vi "VFDRxClearLoop.vi"   [LabVIEW 2018]
uses:
  <vilib>/rvi/DataTransferAndStorage/Container/XNode/niFpgaContainer.xnode
  <vilib>/eio/EIOMethodNode/EIOMethodNode.xnode
  <vilib>/rvi/eio/common/nirviEmuTemplateMethod_errors.vi
  <vilib>/rvi/FIFO/Fifo_Resource/nirvififoEmulationClear.vi
  <vilib>/rvi/FIFO/Fifo_Resource/nirvififoEmulationRead.vi
  <vilib>/rvi/FIFO/Fifo_Resource/nirvififoEmulationWrite.vi
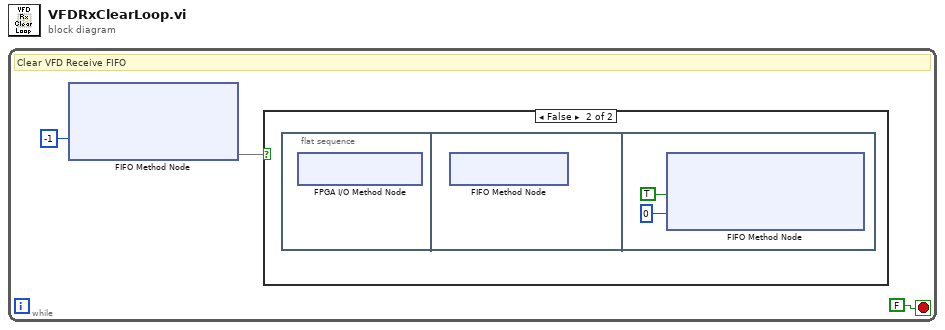
[diagram p0: block diagram]
diagram:
  n1 = while {
    stop <- FALSE stop-if-true
    # "Clear VFD Receive FIFO"
    n2 = xnode ("FIFO Method Node")("Timeout"=-1) -> ("Timed Out?"=w1)  [unwired: 1 in, 2 out]
    n3 = case shown="False" w1 {
      frame True {
      }
      frame False {
        n4 = flat-sequence {
          frame #0 {
            n5 = xnode "FPGA I/O Method Node"() -> ()  [unwired: 1 in, 1 out]
          }
          frame #1 {
            n6 = xnode ("FIFO Method Node")() -> ()  [unwired: 1 in, 1 out]
          }
          frame #2 {
            n7 = xnode ("FIFO Method Node")("Element"=TRUE, "Timeout"=0) -> ()  [unwired: 1 in, 2 out]
          }
        }
      }
    }
  }
